vi "数组创建和替换.vi"() -> ()   [LabVIEW 2018]
panel:
  out "输出数组 3":dbl[][](array[numeric])
  out "输出数组 2":dbl[][](array[numeric])
  out "输出数组":dbl[][](array[numeric])
  out "数组":dbl[][](array[numeric])
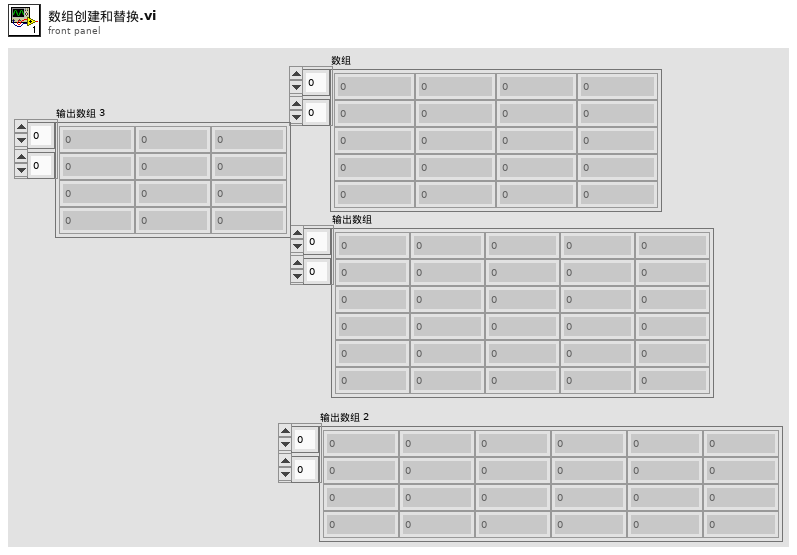
[diagram p1: front panel]
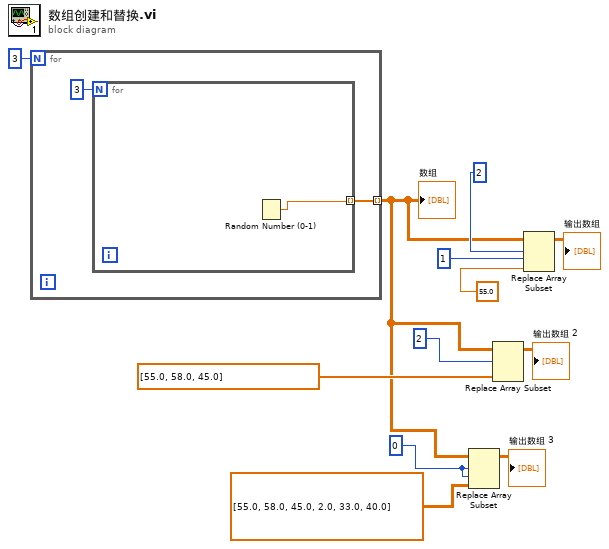
[diagram p0: block diagram]
diagram:
  w1 = 0 ("索引 (行)")
  n1 = for {
    N: 3 -> [_]
    tunnel: [w13] -> w3 mode=indexing
    n2 = for {
      N: 3 -> [_]
      tunnel: [w15] -> w13 mode=indexing
      n3 = Random Number (0-1)() -> (number: 0 to 1=w15:dbl)
    }
  }
  "数组" <- w3
  n4 = Replace Array Subset(array=w3, new element=dbl[][] [[55.0, 58.0, 45.0], [2.0, 33.0, 40.0]] ("新元素/子数组"), index (row)=w1, index (col)=w1) -> (→"输出数组 3":dbl[][])
  n5 = Replace Array Subset(array=w3, new element=dbl[] [55.0, 58.0, 45.0] ("新元素/子数组"), index (row)=2 ("索引 (行)")) -> (→"输出数组 2":dbl[][])  [unwired: 1 in]
  n6 = Replace Array Subset(array=w3, new element=55.0 ("新元素/子数组"), index (row)=2 ("索引 (行)"), index (col)=1 ("禁用的索引 (列)")) -> (→"输出数组":dbl[][])
